vi "Counter U8.vi"(10 "Reset Counter":bool, 11 "Count To":u8) -> (2 "Current Value":u8, 3 "Value Reached":bool)   [LabVIEW 2021, in "Neopixel - FPGA.lvclass"]
doc: "Counts to <b>Count To</b>. <b>Value Reached</b> outputs True once the counter has counted <b>Value</b> times. <b>Current Value</b> outputs the current value of the counter minus 1. The counter will automatically reset itself once it reaches <b>Value</b>. \n\nNote that <b>Current Value</b> will always lag the actual counter value by 1. This makes this counter very useful for iterating through an array or other types of memory that are 0 indexed."
uses:
  Neopixel - FPGA.lvclass
  Neopixel - FPGA.lvclass/Neopixel - FPGA.ctl
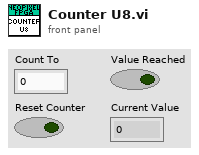
[diagram p1: front panel]
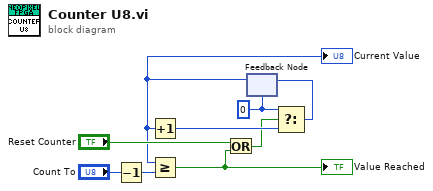
[diagram p0: block diagram]
diagram:
  w8 = u8 0
  n1 = Decrement(x="Count To") -> (x-1=w4:u8)
  n2 = feedback #1(w8) -> (w1:u8)
  "Current Value" <- w1
  n3 = Increment(x=w1) -> (x+1=w9:u8)
  n4 = Greater Or Equal?(x=w1, y=w4) -> (x >= y?=w3:bool)
  "Value Reached" <- w3
  n5 = Or(x="Reset Counter", y=w3) -> (x .or. y?=w7:bool)
  n6 = Select(t=w8, s=w7, f=w9) -> (s? t:f=w2:u8)
  n7 = feedback-in #1(w2) -> ()
